vi "CSM - Set TMO of Sync-Reply.vi"(8 "Error In":errorcluster caption="error in (no error)", 11 "TMO For Sync-Rep (ms) In":i32=5000) -> (0 "error out":errorcluster, 3 "TMO For Sync-Rep (ms) Out":i32=8000)   [LabVIEW 2017, in "Communicable State Machine.lvlib"]
uses:
  Communicable State Machine.lvlib
  _Support/ChangeFlag/FlagInstance-Update CSMKVMap.vi
  _Support/ChangeFlag/ChangeFlag-Write.vi
  Utility/Random Change Flag.vi
  _Support/ChangeFlag/ChangeFlagDB.vi
  _Support/CSMKVMap/CSMKVMapDVR.vi
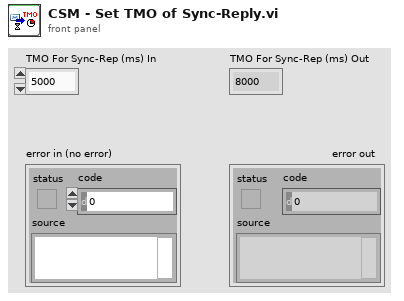
[diagram p1: front panel]
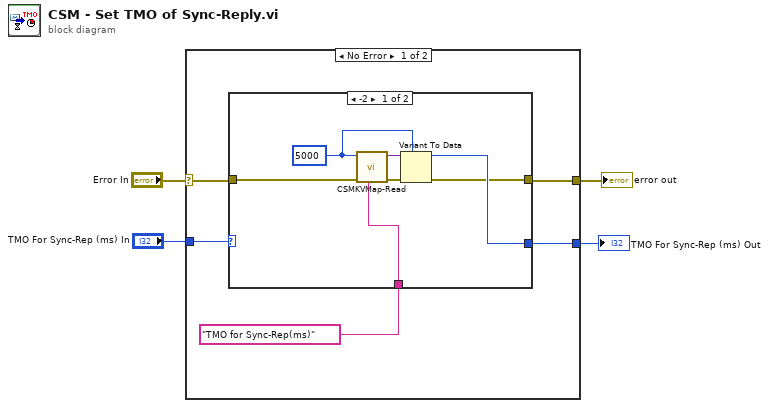
[diagram p0: block diagram]
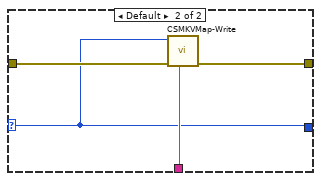
[diagram p2: hidden frame]
diagram:
  n1 = case shown="No Error" "Error In" {
    selector: "Error In" -> [w7 w21]
    tunnel: [w6 w21] -> w3
    tunnel: "TMO For Sync-Rep (ms) In" -> [w9 _]
    tunnel: [w8 _] -> w1
    frame No Error {
      n2 = case shown="-2" w9 {
        selector: w9 -> [_ w17]
        tunnel: [w13 w17] -> w8
        tunnel: [w12 w19] -> w6
        tunnel: w7 -> [w11 w20]
        tunnel: "TMO for Sync-Rep(ms)" ("name") -> [w10 w18]
        frame -2 {
          w14 = 5000 ("max queue size (-1, unlimited)")
          n3 = call "CSMKVMap-Read.vi"("name"=w10, "Error in"=w11, "default value (empty variant)"=w14) -> ("Error out"=w16:errorcluster, "value"=w15:variant)  [unwired: 5 in]
          n4 = Variant To Data(error in=w16, type=w14, Variant=w15) -> (data=w13:i32, error out=w12:errorcluster)
        }
        frame Default {
          n5 = call "CSMKVMap-Write.vi"("name"=w18, "Error in"=w20, "value"=w17) -> ("Error out"=w19:errorcluster)  [unwired: 6 in]
        }
      }
    }
    frame Error {
    }
  }
  "error out" <- w3
  "TMO For Sync-Rep (ms) Out" <- w1
